vi "215.Load Loop 1(SubVI).vi"(0 "VISA multiposition valve":refnum<visa-resource-name>="COM7", 1 "volume":i32=1000, 2 "Syringe Cycle (ms)":u32=1000, 3 "VISA Isolation Valve 2":refnum<visa-resource-name>="COM7", 5 "VISA GILSON":refnum<visa-resource-name>="COM7", 7 "X1 in":i32=1500 min=50 max=5900 step=1, 9 "Y1 in":i32=650 min=50 max=3300 step=1, 11 "error in (no error)":errorcluster, 12 "Double injection":bool) -> (4 "VISA MULTIPOS valve 2":refnum<visa-resource-name>, 6 "VISA out":refnum<visa-resource-name>, 8 "Completed":bool, 10 "String msg":string, 15 "error out":errorcluster)   [LabVIEW 2017]
panel:
  in  "Flush Position":u32=6
  in  "Loop Position":u32=2
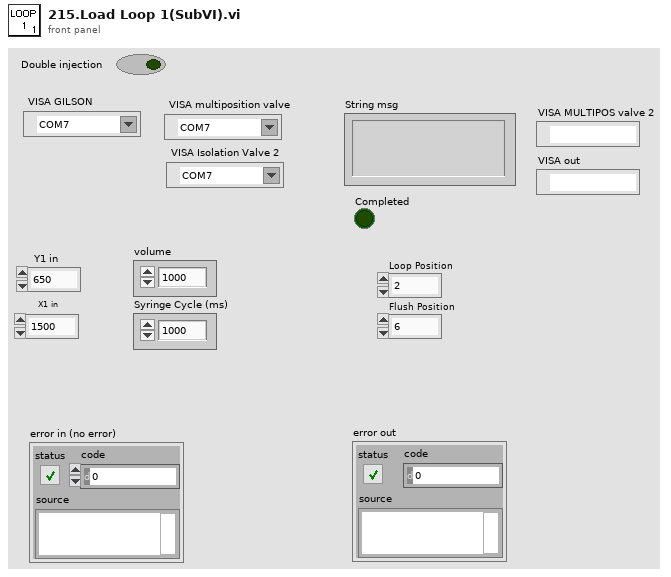
[diagram p1: front panel]
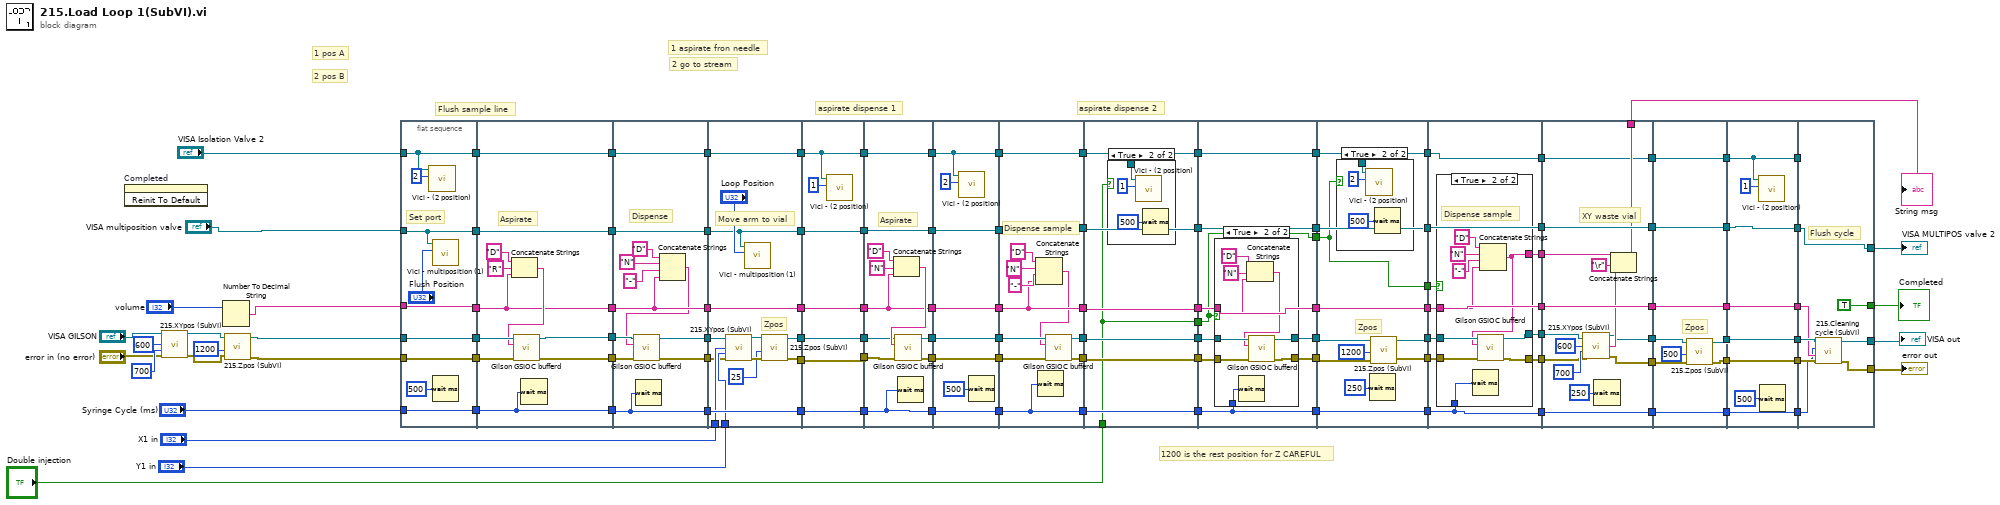
[diagram p0: block diagram]
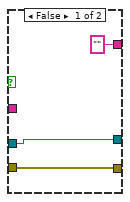
[diagram p5: hidden frame]
diagram:
  # "1200 is the rest position for Z CAREFUL"
  # "2 pos B"
  # "1 pos A"
  # "Flush sample line"
  # "2 go to stream"
  # "1 aspirate fron needle"
  # "aspirate dispense 2"
  # "aspirate dispense 1"
  n1 = invoke on="Completed" class="Bool (strict)" method="Reinit To Default"() -> ()  [unwired: 3 in, 3 out]
  n2 = call "215.XYpos (SubVI).vi"("VISA resource name"="VISA GILSON", "X"=600, "Y"=700, "error in (no error)"="error in (no error)") -> ("VISA Out"=w45:refnum<visa-resource-name>, "error out"=w46:errorcluster)  [unwired: 8 in, 2 out]
  n3 = Number To Decimal String(number="volume") -> (decimal integer string=w96:string)  [unwired: 1 in]
  n4 = call "215.Zpos (SubVI).vi"("error in (no error)"=w46, "Z"=1200, "VISA resource name"=w45) -> ("error out"=w94:errorcluster, "VISA Out"=w95:refnum<visa-resource-name>)  [unwired: 5 in, 2 out]
  n5 = flat-sequence {
    tunnel: [w125] -> w116
    tunnel: w95 -> [w125]
    tunnel: [w124] -> w115
    tunnel: w94 -> [w124]
    tunnel: [w122] -> w114
    tunnel: "Syringe Cycle (ms)" -> [w122]
    tunnel: [w121] -> w113
    tunnel: w96 -> [w121]
    tunnel: "VISA multiposition valve" -> [w120]
    tunnel: [w120] -> w66
    tunnel: "VISA Isolation Valve 2" -> [w117]
    tunnel: [w117] -> w30
    tunnel: w116 -> [w136]
    tunnel: w115 -> [w135]
    tunnel: [w131] -> w38
    tunnel: [w130] -> w39
    tunnel: w114 -> [w129]
    tunnel: [w129] -> w40
    tunnel: w113 -> [w128]
    tunnel: [w128] -> w41
    tunnel: w66 -> [w127]
    tunnel: [w127] -> w37
    tunnel: [w126] -> w31
    tunnel: w30 -> [w126]
    tunnel: [w148] -> w60
    tunnel: [w147] -> w58
    tunnel: w41 -> [w147]
    tunnel: w40 -> [w148]
    tunnel: w39 -> [w144]
    tunnel: w38 -> [w145]
    tunnel: [w140] -> w54
    tunnel: w37 -> [w140]
    tunnel: [w139] -> w50
    tunnel: [w138] -> w49
    tunnel: [w137] -> w32
    tunnel: w31 -> [w137]
    tunnel: w60 -> [w162]
    tunnel: [w162] -> w59
    tunnel: w58 -> [w152]
    tunnel: [w152] -> w57
    tunnel: [w154] -> w56
    tunnel: [w153] -> w55
    tunnel: w54 -> [w149]
    tunnel: [w149] -> w53
    tunnel: "X1 in" -> [w158]
    tunnel: "Y1 in" -> [w157]
    tunnel: w50 -> [w156]
    tunnel: w49 -> [w155]
    tunnel: [w151] -> w33
    tunnel: w32 -> [w151]
    tunnel: [w166] -> w112
    tunnel: [w169] -> w111
    tunnel: w59 -> [w169]
    tunnel: w57 -> [w168]
    tunnel: [w168] -> w110
    tunnel: [w167] -> w109
    tunnel: w56 -> [w167]
    tunnel: w55 -> [w166]
    tunnel: w53 -> [w165]
    tunnel: [w165] -> w65
    tunnel: [w163] -> w34
    tunnel: w33 -> [w163]
    tunnel: w112 -> [w179]
    tunnel: [w176] -> w88
    tunnel: [w175] -> w87
    tunnel: w111 -> [w174]
    tunnel: [w174] -> w86
    tunnel: w110 -> [w173]
    tunnel: [w173] -> w85
    tunnel: w109 -> [w172]
    tunnel: w65 -> [w171]
    tunnel: [w171] -> w64
    tunnel: [w170] -> w35
    tunnel: w34 -> [w170]
    tunnel: w88 -> [w188]
    tunnel: [w188] -> w84
    tunnel: w87 -> [w187]
    tunnel: [w187] -> w83
    tunnel: w86 -> [w186]
    tunnel: [w186] -> w82
    tunnel: w85 -> [w185]
    tunnel: [w185] -> w81
    tunnel: w64 -> [w183]
    tunnel: [w183] -> w63
    tunnel: w35 -> [w181]
    tunnel: [w181] -> w25
    tunnel: w84 -> [w196]
    tunnel: [w193] -> w80
    tunnel: w83 -> [w195]
    tunnel: w82 -> [w192]
    tunnel: [w192] -> w79
    tunnel: w81 -> [w197]
    tunnel: [w197] -> w78
    tunnel: [w194] -> w77
    tunnel: w63 -> [w190]
    tunnel: [w190] -> w62
    tunnel: [w189] -> w26
    tunnel: w25 -> [w189]
    tunnel: [w203] -> w76
    tunnel: w80 -> [w207]
    tunnel: [w207] -> w74
    tunnel: [w206] -> w72
    tunnel: w79 -> [w205]
    tunnel: [w205] -> w70
    tunnel: w78 -> [w204]
    tunnel: [w204] -> w68
    tunnel: w77 -> [w206]
    tunnel: w62 -> [w203]
    tunnel: [w202] -> w27
    tunnel: w26 -> [w202]
    tunnel: [w201] -> w22
    tunnel: "Double injection" -> [w201]
    tunnel: w76 -> [w219]
    tunnel: [w219] -> w75
    tunnel: w74 -> [w214]
    tunnel: [w215] -> w73
    tunnel: w72 -> [w217]
    tunnel: [w216] -> w71
    tunnel: w70 -> [w213]
    tunnel: [w213] -> w69
    tunnel: w68 -> [w218]
    tunnel: [w218] -> w67
    tunnel: [w212] -> w28
    tunnel: w27 -> [w212]
    tunnel: w22 -> [w211]
    tunnel: [w211] -> w20
    tunnel: w75 -> [w234]
    tunnel: w73 -> [w235]
    tunnel: w71 -> [w236]
    tunnel: [w237] -> w106
    tunnel: [w241] -> w107
    tunnel: w69 -> [w241]
    tunnel: [w240] -> w108
    tunnel: w67 -> [w240]
    tunnel: [w238] -> w105
    tunnel: [w234] -> w104
    tunnel: [w233] -> w29
    tunnel: w28 -> [w233]
    tunnel: [w232] -> w23
    tunnel: w20 -> [w232]
    tunnel: [w254] -> w14
    tunnel: [w253] -> w13
    tunnel: w108 -> [w254]
    tunnel: w107 -> [w253]
    tunnel: w106 -> [w251]
    tunnel: w105 -> [w252]
    tunnel: w104 -> [w250]
    tunnel: [w250] -> w15
    tunnel: [w249] -> w16
    tunnel: [w248] -> w17
    tunnel: [w247] -> w18
    tunnel: w29 -> [w246]
    tunnel: [w246] -> w19
    tunnel: w23 -> [w245]
    tunnel: [w282] -> w12
    tunnel: [w281] -> w10
    tunnel: [w280] -> w6
    tunnel: [w274] -> w42
    tunnel: [w273] -> w4
    tunnel: [w272] -> w2
    tunnel: [w271] -> w1
    tunnel: w13 -> [w282]
    tunnel: w14 -> [w281]
    tunnel: w15 -> [w280]
    tunnel: w16 -> [w269]
    tunnel: w17 -> [w270]
    tunnel: w18 -> [w275]
    tunnel: w19 -> [w273]
    tunnel: w12 -> [w291]
    tunnel: [w291] -> w11
    tunnel: w10 -> [w290]
    tunnel: [w290] -> w9
    tunnel: [w283] -> w8
    tunnel: [w284] -> w7
    tunnel: w6 -> [w289]
    tunnel: [w289] -> w5
    tunnel: w4 -> [w288]
    tunnel: [w288] -> w3
    tunnel: w2 -> [w286]
    tunnel: w1 -> [w285]
    tunnel: w11 -> [w299]
    tunnel: [w299] -> w103
    tunnel: w9 -> [w298]
    tunnel: [w298] -> w102
    tunnel: w8 -> [w297]
    tunnel: [w297] -> w101
    tunnel: w7 -> [w296]
    tunnel: [w296] -> w100
    tunnel: w5 -> [w294]
    tunnel: [w294] -> w90
    tunnel: w3 -> [w292]
    tunnel: [w292] -> w24
    tunnel: w103 -> [w304]
    tunnel: w102 -> [w305]
    tunnel: w101 -> [w306]
    tunnel: w100 -> [w307]
    tunnel: [TRUE] -> w93
    tunnel: [w302] -> w92
    tunnel: [w301] -> w91
    tunnel: [w300] -> w89
    tunnel: w90 -> [w300]
    tunnel: w24 -> [_]
    frame #0 {
      # "Set port"
      n6 = call "Vici - (2 position).vi"("Position"=u32 2, "VISA resource name"=w117) -> ()  [unwired: 10 in]
      n7 = call "Vici - multiposition (1).vi"("Position"="Flush Position", "VISA resource name"=w120) -> ()  [unwired: 9 in, 1 out]
      n8 = Wait (ms)(milliseconds to wait=u32 500) -> ()  [unwired: 1 out]
    }
    frame #1 {
      # "Aspirate"
      n9 = Concatenate Strings("D" ("string"), "R" ("string"), w128) -> (w132:string)
      n10 = call <instrlib>:"Gilson GSIOC bufferd.vi"("error in (no error)"=w135, "Bufferd command"=w132, "VISA resource name"=w136) -> ("error out"=w130:errorcluster, "VISA resource name out"=w131:refnum<visa-resource-name>)  [unwired: 6 in, 1 out]
      n11 = Wait (ms)(milliseconds to wait=w129) -> ()  [unwired: 1 out]
    }
    frame #2 {
      # "Dispense"
      n12 = Wait (ms)(milliseconds to wait=w148) -> ()  [unwired: 1 out]
      n13 = Concatenate Strings("D" ("string"), "N" ("string"), "-" ("string"), w147) -> (w141:string)
      n14 = call <instrlib>:"Gilson GSIOC bufferd.vi"("error in (no error)"=w144, "Bufferd command"=w141, "VISA resource name"=w145) -> ("error out"=w139:errorcluster, "VISA resource name out"=w138:refnum<visa-resource-name>)  [unwired: 6 in, 1 out]
    }
    frame #3 {
      # "Move arm to vial"
      # "Zpos"
      n15 = call "215.XYpos (SubVI).vi"("VISA resource name"=w155, "X"=w158, "Y"=w157, "error in (no error)"=w156) -> ("VISA Out"=w161:refnum<visa-resource-name>, "error out"=w160:errorcluster)  [unwired: 8 in, 2 out]
      n16 = call "Vici - multiposition (1).vi"("Position"="Loop Position", "VISA resource name"=w149) -> ()  [unwired: 9 in, 1 out]
      n17 = call "215.Zpos (SubVI).vi"("error in (no error)"=w160, "Z"=25, "VISA resource name"=w161) -> ("error out"=w153:errorcluster, "VISA Out"=w154:refnum<visa-resource-name>)  [unwired: 5 in, 2 out]
    }
    frame #4 {
      n18 = call "Vici - (2 position).vi"("Position"=u32 1, "VISA resource name"=w163) -> ()  [unwired: 10 in]
    }
    frame #5 {
      # "Aspirate"
      n19 = Concatenate Strings("D" ("string"), "N" ("string"), w173) -> (w177:string)
      n20 = call <instrlib>:"Gilson GSIOC bufferd.vi"("error in (no error)"=w179, "Bufferd command"=w177, "VISA resource name"=w172) -> ("error out"=w176:errorcluster, "VISA resource name out"=w175:refnum<visa-resource-name>)  [unwired: 6 in, 1 out]
      n21 = Wait (ms)(milliseconds to wait=w174) -> ()  [unwired: 1 out]
    }
    frame #6 {
      n22 = call "Vici - (2 position).vi"("Position"=u32 2, "VISA resource name"=w181) -> ()  [unwired: 10 in]
      n23 = Wait (ms)(milliseconds to wait=u32 500) -> ()  [unwired: 1 out]
    }
    frame #7 {
      # "Dispense sample"
      n24 = Concatenate Strings("D" ("string"), "N" ("string"), "-" ("string"), w197) -> (w191:string)
      n25 = Wait (ms)(milliseconds to wait=w192) -> ()  [unwired: 1 out]
      n26 = call <instrlib>:"Gilson GSIOC bufferd.vi"("error in (no error)"=w196, "Bufferd command"=w191, "VISA resource name"=w195) -> ("error out"=w193:errorcluster, "VISA resource name out"=w194:refnum<visa-resource-name>)  [unwired: 6 in, 1 out]
    }
    frame #8 {
      n27 = case shown="True" w201 {
        tunnel: w202 -> [_ w209]
        frame False {
        }
        frame True {
          n28 = call "Vici - (2 position).vi"("Position"=u32 1, "VISA resource name"=w209) -> ()  [unwired: 10 in]
          n29 = Wait (ms)(milliseconds to wait=u32 500) -> ()  [unwired: 1 out]
        }
      }
    }
    frame #9 {
      n30 = case shown="True" w211 {
        tunnel: w218 -> [_ w228]
        tunnel: w217 -> [w221 w227]
        tunnel: [w221 w226] -> w216
        tunnel: [w220 w225] -> w215
        tunnel: w214 -> [w220 w224]
        tunnel: w213 -> [_ w222]
        frame False {
        }
        frame True {
          n31 = Wait (ms)(milliseconds to wait=w222) -> ()  [unwired: 1 out]
          n32 = Concatenate Strings("D" ("string"), "N" ("string"), w228) -> (w223:string)
          n33 = call <instrlib>:"Gilson GSIOC bufferd.vi"("error in (no error)"=w224, "Bufferd command"=w223, "VISA resource name"=w227) -> ("error out"=w225:errorcluster, "VISA resource name out"=w226:refnum<visa-resource-name>)  [unwired: 6 in, 1 out]
        }
      }
    }
    frame #10 {
      # "Zpos"
      n34 = case shown="True" w232 {
        tunnel: w233 -> [_ w243]
        frame False {
        }
        frame True {
          n35 = call "Vici - (2 position).vi"("Position"=u32 2, "VISA resource name"=w243) -> ()  [unwired: 10 in]
          n36 = Wait (ms)(milliseconds to wait=u32 500) -> ()  [unwired: 1 out]
        }
      }
      n37 = Wait (ms)(milliseconds to wait=u32 250) -> ()  [unwired: 1 out]
      n38 = call "215.Zpos (SubVI).vi"("error in (no error)"=w235, "Z"=1200, "VISA resource name"=w236) -> ("error out"=w238:errorcluster, "VISA Out"=w237:refnum<visa-resource-name>)  [unwired: 5 in, 2 out]
    }
    frame #11 {
      n39 = case shown="True" w245 {
        tunnel: w254 -> [_ w267]
        tunnel: w253 -> [_ w266]
        tunnel: w252 -> [w256 w263]
        tunnel: w251 -> [w257 w262]
        tunnel: [w257 w260] -> w249
        tunnel: [w256 w259] -> w248
        tunnel: ["" w258] -> w247
        frame False {
        }
        frame True {
          # "Dispense sample"
          n40 = Wait (ms)(milliseconds to wait=w266) -> ()  [unwired: 1 out]
          n41 = Concatenate Strings("D" ("string"), "N" ("string"), "-" ("string"), w267) -> (w258:string)
          n42 = call <instrlib>:"Gilson GSIOC bufferd.vi"("error in (no error)"=w263, "Bufferd command"=w258, "VISA resource name"=w262) -> ("error out"=w259:errorcluster, "VISA resource name out"=w260:refnum<visa-resource-name>)  [unwired: 6 in, 1 out]
        }
      }
    }
    frame #12 {
      # "XY waste vial"
      n43 = call "215.XYpos (SubVI).vi"("VISA resource name"=w269, "X"=600, "Y"=700, "error in (no error)"=w270) -> ("VISA Out"=w271:refnum<visa-resource-name>, "Receive string"=w276:string, "error out"=w272:errorcluster)  [unwired: 8 in, 1 out]
      n44 = Wait (ms)(milliseconds to wait=u32 250) -> ()  [unwired: 1 out]
      n45 = Concatenate Strings(w275, "\r", w276) -> (w274:string)
    }
    frame #13 {
      # "Zpos"
      n46 = call "215.Zpos (SubVI).vi"("error in (no error)"=w286, "Z"=500, "VISA resource name"=w285) -> ("error out"=w283:errorcluster, "VISA Out"=w284:refnum<visa-resource-name>)  [unwired: 5 in, 2 out]
    }
    frame #14 {
      n47 = call "Vici - (2 position).vi"("Position"=u32 1, "VISA resource name"=w292) -> ()  [unwired: 10 in]
      n48 = Wait (ms)(milliseconds to wait=u32 500) -> ()  [unwired: 1 out]
    }
    frame #15 {
      # "Flush cycle"
      n49 = call "215.Cleaning cycle (SubVI).vi"("error in (no error)"=w306, "Volumen (-1000 to 0)"=w305, "milliseconds to wait"=w304, "VISA Refnum in"=w307) -> ("error out"=w302:errorcluster, "VISA out"=w301:refnum<visa-resource-name>)  [unwired: 5 in, 1 out]
    }
  }
  "String msg" <- w42
  "Completed" <- w93
  "error out" <- w92
  "VISA out" <- w91
  "VISA MULTIPOS valve 2" <- w89
